vi "Menu Set Enable.vi"(8 "error in (no error)":errorcluster, 10 "enabled ?":bool, 11 "Menu in":refnum<k9>) -> (0 "error out":errorcluster, 3 "Menu out":refnum<k9>)   [LabVIEW 2019, in "CML UI.lvlib"]
uses:
  CML UI.lvlib
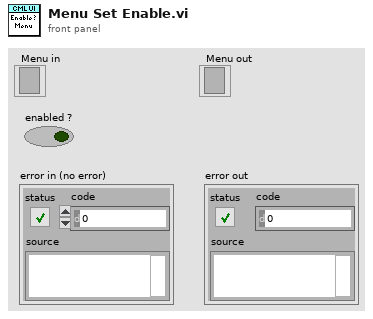
[diagram p1: front panel]
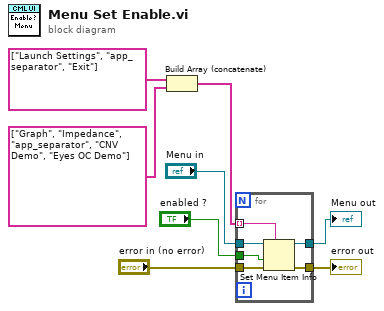
[diagram p0: block diagram]
diagram:
  n1 = Build Array (concatenate)(string[] ["Launch Settings", "app_separator", "Exit"] ("L10n_item tags 2"), string[] ["Graph", "Impedance", "app_separator", "CNV Demo", "Eyes OC Demo"] ("L10n_item tags 2")) -> (w5:string[])
  n2 = for {
    tunnel: "enabled ?" -> [w14]
    tunnel: "Menu in" -> [w13]
    tunnel: w5 -> [w12] mode=indexing
    tunnel: [w11] -> w6
    tunnel: "error in (no error)" -> [w10]
    tunnel: [w9] -> w8
    n3 = Set Menu Item Info(7:w12, 8:w10, 9:w14, 11:w13) -> (0:w9:errorcluster, 3:w11:refnum<k9>)  [unwired: 3 in]
  }
  "Menu out" <- w6
  "error out" <- w8
